vi "Prepare State.vi"(8 "error in (no error)":errorcluster, 10 "Context in":refnum<class "State Pattern.lvclass">) -> (0 "error out":errorcluster, 3 "State out":refnum<class "State Pattern.lvclass">, 5 "Context out (for Preserve Run-Time Class)":refnum<class "State Pattern.lvclass">)   [LabVIEW 2021, in "State Pattern.lvclass"]
uses:
  State Pattern.lvclass
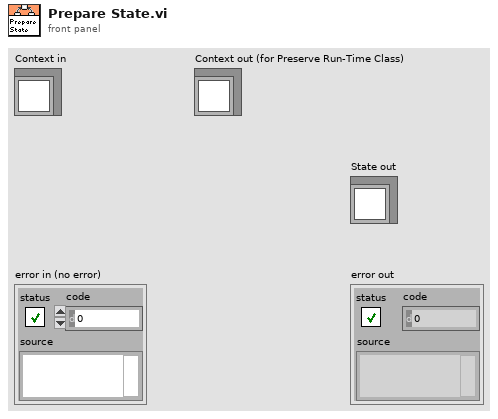
[diagram p1: front panel]
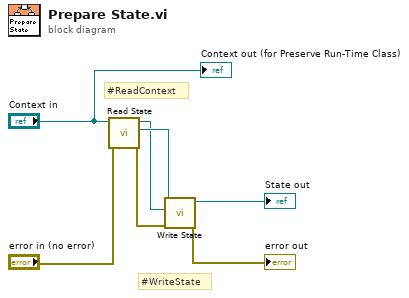
[diagram p0: block diagram]
diagram:
  # "#WriteState"
  # "#ReadContext"
  n1 = call-dynamic "Read State.vi"("error in (no error)"="error in (no error)", "State Pattern in"="Context in") -> ("error out"=w7:errorcluster, "State"=w6:refnum<class "State Pattern.lvclass">, "State Pattern out"=w5:refnum<class "State Pattern.lvclass">)  [unwired: 7 in]
  n2 = call-dynamic "Write State.vi"("error in (no error)"=w7, "State"=w5, "State Pattern in"=w6) -> ("error out"=→"error out":errorcluster, "State Pattern out"=→"State out":refnum<class "State Pattern.lvclass">)  [unwired: 7 in]
  "Context out (for Preserve Run-Time Class)" <- "Context in"
